vi "LS 336 T Ramp Com.vi"(2 "command text in":string[](array[string]), 3 "option":T2) -> (1 "Command text out":string[][](array[string]))   [LabVIEW 2024]
uses:
  Ctl/option.ctl
  LS 336 T Ramp.ctl
panel:
  in  "Timed Ramp":T1={"VISA Resource Name"="", "extra wait"=1, "start"=1e-12, "end"=0.002, "Sweep Time (H:M:S)"=1800.0, "Log Linear"=FALSE, "Heater Range"=enum."OFF", "Loop"=FALSE} {"Sweep Time (H:M:S)" format="%<%H:%M:%S>t"; "extra wait" min=0; "start" format="%#.7e"; "end" format="%#.7e"}
  in  "enter":bool
  in  "cancel":bool
  # "LS 336 Temp Setpoint (K) Ramp"
  # "Log"
  # "End Temp (K)"
  # "Sweep Time (HH:MM:SS)"
  # "Start Temp (K)"
  # "Linear"
  # "seconds"
  # "AND wait extra"
  # "Which Heater to control?"
  # "VISA Name"
  # "Loop 2\n(Probe / 3He Pot)"
  # "Heater Range"
  # "Loop 1\n(Sorb / VTI)"
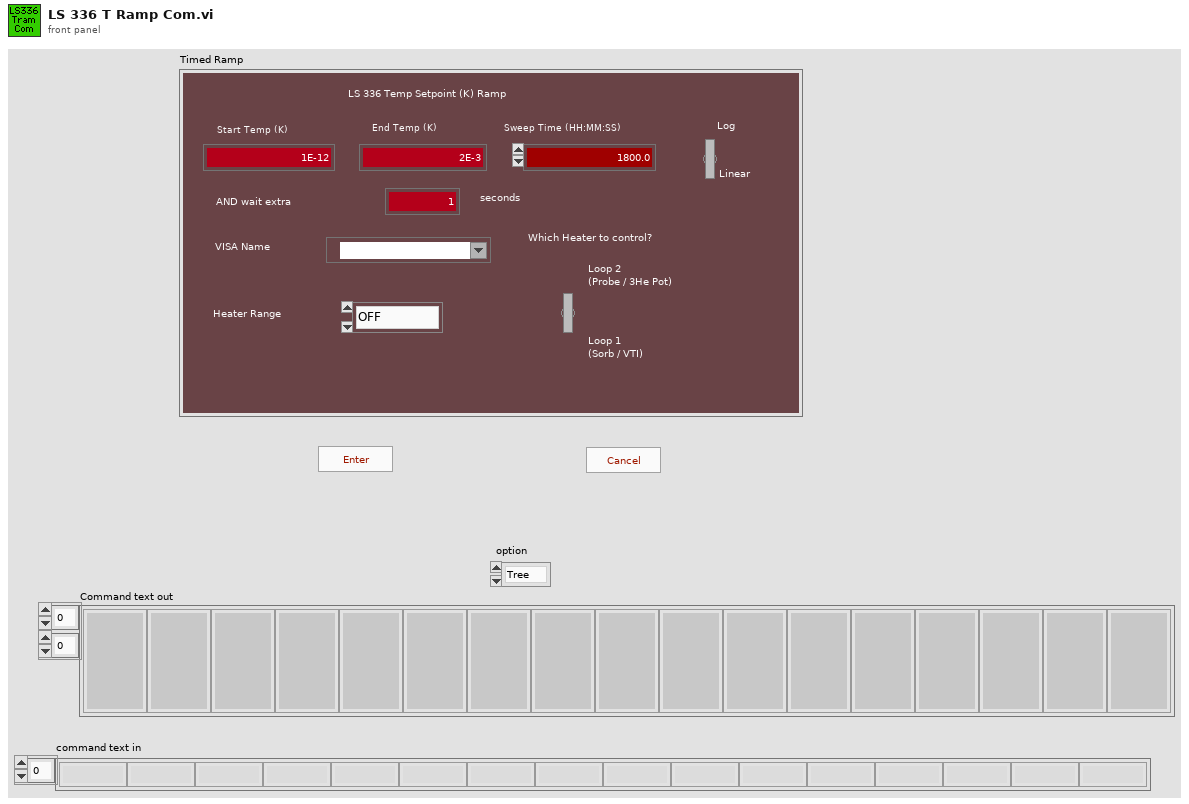
[diagram p1: front panel]
types:
  T1 = typedef "LS 336 T Ramp.ctl" = cluster{"VISA Resource Name":refnum<visa-resource-name>, "extra wait":i32, "start":dbl, "end":dbl, "Sweep Time (H:M:S)":dbl, "Log Linear":bool, "Heater Range":enum16{"OFF", "LOW", "MEIDUM", "HIGH"}, "Loop":bool}
  T2 = typedef "option.ctl" = enum16{"Tree", "List"}
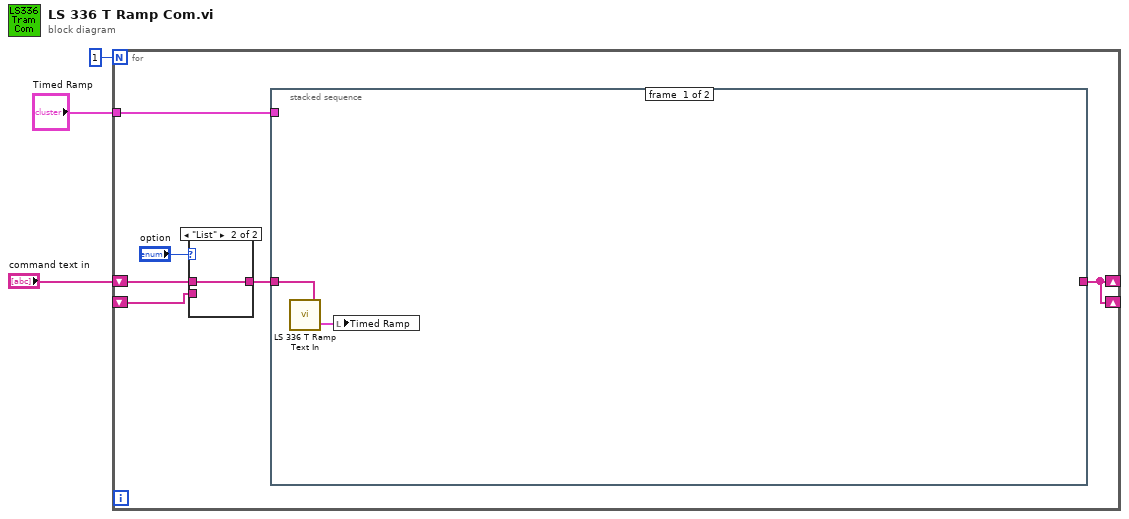
[diagram p0: block diagram]
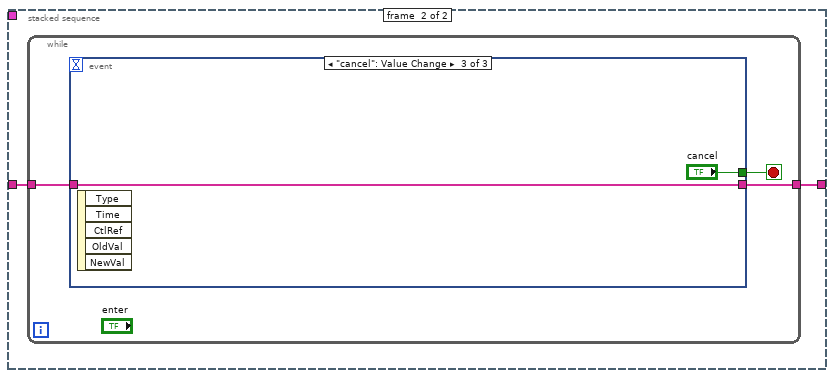
[diagram p3: hidden frame]
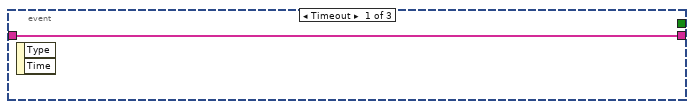
[diagram p4: hidden frame]
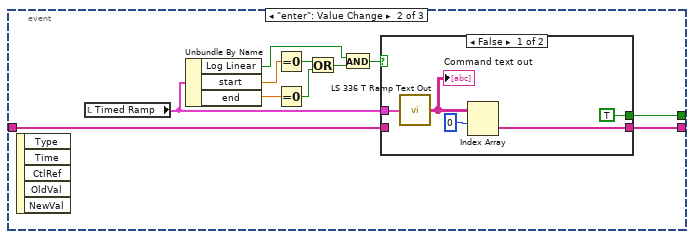
[diagram p5: hidden frame]
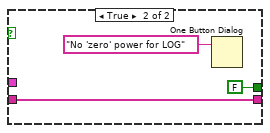
[diagram p6: hidden frame]
diagram:
  n1 = for {
    N: 1 -> [_]
    shift-right: [w6] -> _
    shift-left: _ -> [w8]
    shift-right: [w6] -> _
    shift-left: "command text in" -> [w7]
    tunnel: "Timed Ramp" -> [w4]
    n2 = case shown="\"List\"" "option" {
      tunnel: [w10 w11] -> w9
      tunnel: w8 -> [w10 _]
      tunnel: w7 -> [_ w11]
      frame "Tree", Default {
      }
      frame "List" {
      }
    }
    n3 = stacked-sequence {
      tunnel: [_ w15] -> w6
      tunnel: w9 -> [w13 w14]
      tunnel: w4 -> [_ _]
      frame #0 {
        n4 = call "LS 336 T Ramp Text In.vi"("command text in"=w13) -> ("Timed Ramp"=w12:T1)  [unwired: 4 in]
        n5 = local write "Timed Ramp"(w12) -> ()
      }
      frame #1 {
        n6 = while {
          tunnel: [w17] -> w15
          tunnel: w14 -> [w16]
          stop <- w18 stop-if-true
          n7 = event shown="[2] \"cancel\": Value Change" {
            selector: _ -> [_ _ _]
            dyn-events: _ -> [_ _ _]
            timeout: _ -> [_ _ _]
            tunnel: [_ w20 "cancel"] -> w18
            tunnel: [w19 w30 w39] -> w17
            tunnel: w16 -> [w19 w21 w39]
            event Timeout {
              n8 = event-data() -> ()  [unwired: 1 in, 2 out]
            }
            event "enter": Value Change {
              n9 = event-data() -> ()  [unwired: 1 in, 5 out]
              n10 = local read "Timed Ramp"() -> (w29:T1)
              n11 = Unbundle By Name(w29) -> ("Log Linear"=w24:bool, "start"=w27:dbl, "end"=w26:dbl)
              n12 = Equal To 0?(x=w27) -> (x = 0?=w28:bool)
              n13 = Equal To 0?(x=w26) -> (x = 0?=w25:bool)
              n14 = Or(x=w28, y=w25) -> (x .or. y?=w23:bool)
              n15 = And(x=w24, y=w23) -> (x .and. y?=w22:bool)
              n16 = case shown="False" w22 {
                tunnel: [w33 w38] -> w30
                tunnel: w29 -> [w32 _]
                tunnel: w21 -> [_ w38]
                tunnel: [TRUE FALSE] -> w20
                frame False {
                  n17 = call "LS 336 T Ramp Text Out.vi"("Timed Ramp"=w32) -> ("Command text"=w35:string[][])
                  "Command text out" <- w35
                  n18 = Index Array(array=w35, index (row)=0) -> (element=w33:string[])  [unwired: 1 in]
                }
                frame True {
                  n19 = One Button Dialog(message="No 'zero' power for LOG") -> ()  [unwired: 1 in, 1 out]
                }
              }
            }
            event "cancel": Value Change {
              n20 = event-data() -> ()  [unwired: 1 in, 5 out]
            }
          }
        }
      }
    }
  }
